vi "Check for OOB Commands.vi"(8 "error in (no error)":errorcluster, 11 "CoreOOB_Rx in":refnum<class "TemplateOOB_Rx.lvclass">) -> (0 "error out":errorcluster, 1 "Commands":T1[](array[typedef]), 2 "New Commands":bool, 3 "CoreOOB_Rx out":refnum<class "TemplateOOB_Rx.lvclass">)   [LabVIEW 2021, in "TemplateOOB_Rx.lvclass"]
uses:
  TemplateOOB_Rx.lvclass
  C:/Program Files/National Instruments/LabVIEW 2021/vi.lib/CIF Foundation/CIF Out of Band Commands/CIFOutOfBand.lvclass
  Typedef/OOB Commands.ctl
  <vilib>/CIF Foundation/CIF Out of Band Commands/CIFOutOfBand.lvclass/CIFOutOfBand.ctl
  <vilib>/CIF Foundation/CIF Out of Band Commands/CIFOutOfBand.lvclass
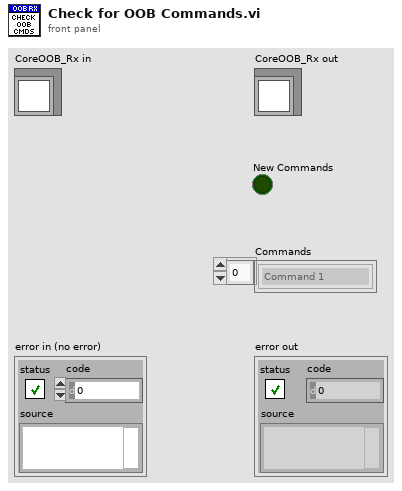
[diagram p1: front panel]
types:
  T1 = typedef "TemplateOOB_Rx.lvclass/OOB Commands.ctl" = enum8{"Command 1"}
  T2 = typedef "TemplateOOB_Rx.lvclass/Command Setting Control.ctl" = cluster{"Enum":T1, "U8":u8, " Payload":bool}
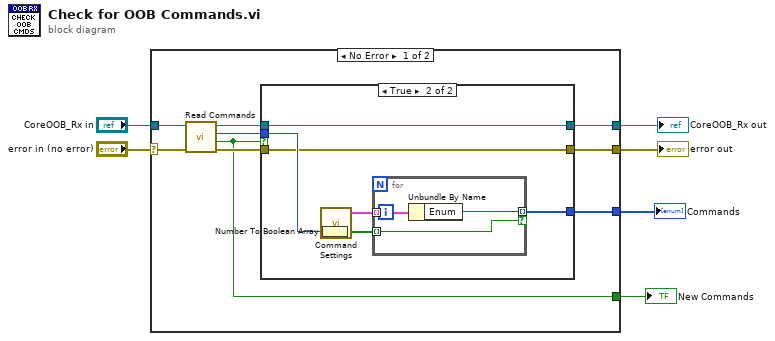
[diagram p0: block diagram]
diagram:
  n1 = case shown="No Error" "error in (no error)" {
    selector: "error in (no error)" -> [w14 w28]
    tunnel: [w9 w28] -> w5
    tunnel: [w10 w27] -> w3
    tunnel: "CoreOOB_Rx in" -> [w15 w27]
    tunnel: [w11 _] -> w2
    tunnel: [w8 _] -> w1
    frame No Error {
      n2 = call <vilib>:"Read Commands.vi"("error in"=w14, "OOB in"=w15) -> ("error out"=w12:errorcluster, "New Commands"=w8:bool, "Commands (bitwise)"=w7:u64, "OOB out"=w13:refnum<class "TemplateOOB_Rx.lvclass">)  [unwired: 6 in]
      n3 = case shown="True" w8 {
        tunnel: w13 -> [w17 w18]
        tunnel: w12 -> [w16 w19]
        tunnel: [_ w21] -> w11
        tunnel: [w17 w18] -> w10
        tunnel: [w16 w19] -> w9
        tunnel: w7 -> [_ w20]
        frame False {
        }
        frame True {
          n4 = Number To Boolean Array(number=w20) -> (Boolean array=w23:bool[])
          n5 = call "Command Settings.vi"() -> ("Command Settings"=w22:T2[])  [unwired: 5 in]
          n6 = for {
            tunnel: w23 -> [w24] mode=indexing
            tunnel: w22 -> [w26] mode=indexing
            tunnel: [w25] -> w21 mode=indexing if=w24
            n7 = Unbundle By Name(w26) -> ("Enum"=w25:T1)
          }
        }
      }
    }
    frame Error {
    }
  }
  "error out" <- w5
  "CoreOOB_Rx out" <- w3
  "Commands" <- w2
  "New Commands" <- w1
